vi "Create.vi"(8 "error in (no error)":errorcluster, 9 "Destination Class Path":path, 10 "Source Class Path":path) -> (0 "error out":errorcluster, 3 "Mock Class Generator Out":refnum<class "Mock Class Generator.lvclass">)   [LabVIEW 2020, in "Mock Class Generator.lvclass"]
uses:
  Mock Class Generator.lvclass
  Mock Class Generator.lvclass/Mock Class Generator.ctl
  <vilib>/Utility/error.llb/Error Cluster From Error Code.vi
  <vilib>/ErrorRing/Error Ring.xnode
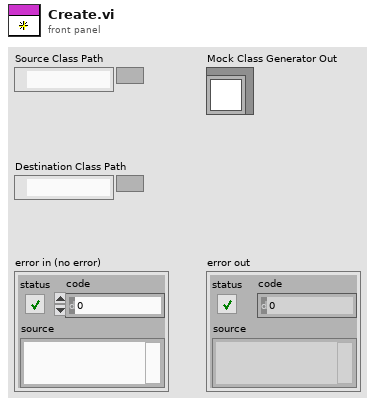
[diagram p1: front panel]
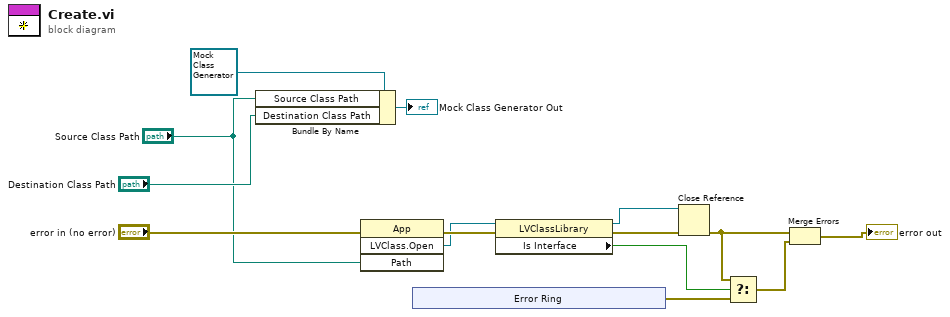
[diagram p0: block diagram]
diagram:
  n1 = Bundle By Name(cluster=refnum<class "Mock Class Generator.lvclass"> refnum ("Mock Class Generator.lvclass"), "Source Class Path"="Source Class Path", "Destination Class Path"="Destination Class Path") -> (→"Mock Class Generator Out":refnum<class "Mock Class Generator.lvclass">)
  n2 = invoke class="App" method="LVClass.Open"(error in="error in (no error)", "Path"="Source Class Path") -> (error out=w10:errorcluster, "LVClass.Open"=w7:refnum<vi>)  [unwired: 2 in, 2 out]
  n3 = xnode "Error Ring"() -> ("error out"=w2:errorcluster)
  n4 = property class="LVClassLibrary"(reference=w7, error in=w10) -> (reference out=w6:refnum<vi>, error out=w8:errorcluster, "Is Interface"=w1:bool)
  n5 = Close Reference(reference=w6, error in (no error)=w8) -> (error out=w4:errorcluster)
  n6 = Select(t=w4, s=w1, f=w2) -> (s? t:f=w3:errorcluster)
  n7 = Merge Errors(w4, w3) -> (→"error out":errorcluster)
